vi "StartCamera.vi"(11 "WebCamViewerRef":refnum<k24>) -> (3 "GetCameras":string[](array[string]))   [LabVIEW 2020]
uses:
  C:/Projects/DXFViewer/LabviewDXFViewer/LabviewDXFViewer/bin/Release/LabviewDXFViewer.exe
  LabviewDXFViewer/bin/Release/LabviewDXFViewer.exe
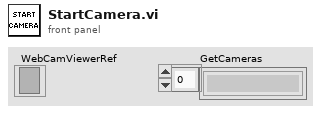
[diagram p1: front panel]
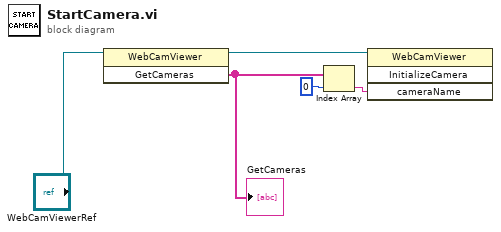
[diagram p0: block diagram]
diagram:
  n1 = invoke class="WebCamViewer" method="GetCameras"(reference="WebCamViewerRef") -> (reference out=w1:refnum<k24>, "GetCameras"=w3:string[])  [unwired: 2 in, 1 out]
  "GetCameras" <- w3
  n2 = Index Array(array=w3, index=0) -> (element=w2:string)
  n3 = invoke class="WebCamViewer" method="InitializeCamera"(reference=w1, "cameraName"=w2) -> ()  [unwired: 2 in, 4 out]
